vi "Mutex Attr Set Priority Ceiling.vi"(8 "error in (no error)":errorcluster, 10 "priority ceiling":i32, 11 "Mutex Attr in":T1) -> (0 "error out":errorcluster, 3 "Mutex Attr out":T1)   [LabVIEW 2013, in "Linux RT IPC.lvlib" / "POSIX Threads.lvlib" / "Mutex Attr.lvclass"]
doc: "Calls pthread_mutexattr_setprioceling() on the pthread mutex attribute object encapsulated by Mutex Attr.\n\nThis VI sets the priority ceiling for the provided mutex attribute object. The priority ceiling refers to the maximum priority that the mutex can be elevated to in the event of a priority inversion.\n\nRefer to online POSIX documentation for more information."
uses:
  Mutex Attr.lvclass
  Controls/reference.ctl
  POSIX Thread Object/POSIX Thread Object.lvclass/POSIX Thread Object.ctl
  POSIX Thread Object/Private VIs/libpthread path.vi
  POSIX Thread Object/Private VIs/get pthread error.vi
  POSIX Thread Object/POSIX Thread Object.lvclass
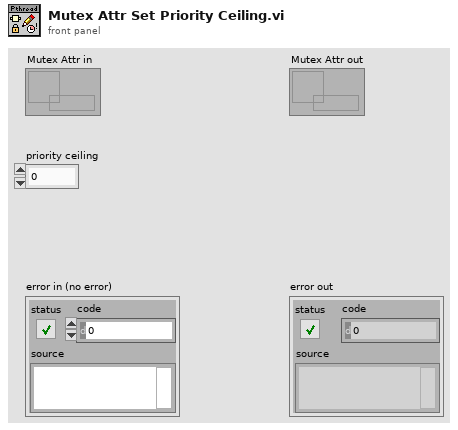
[diagram p1: front panel]
types:
  T1 = typedef "Linux RT IPC.lvlib/POSIX Threads.lvlib/Mutex Attr.lvclass/reference.ctl" = refnum<data-value>
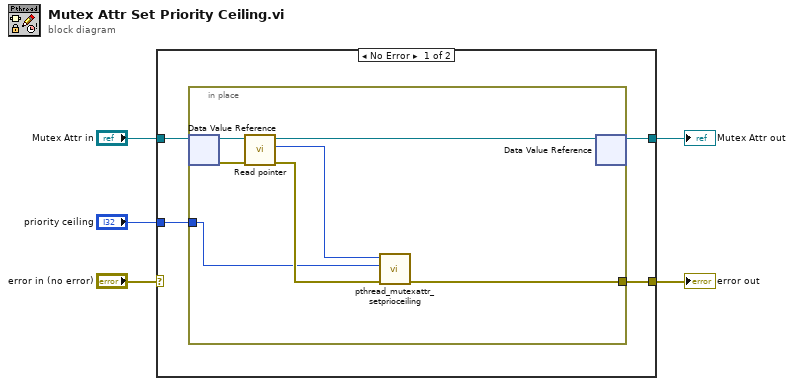
[diagram p0: block diagram]
diagram:
  n1 = case shown="No Error" "error in (no error)" {
    selector: "error in (no error)" -> [_ w18]
    tunnel: [w7 w18] -> w4
    tunnel: "Mutex Attr in" -> [w9 w17]
    tunnel: [w8 w17] -> w2
    tunnel: "priority ceiling" -> [w6 _]
    frame No Error {
      n2 = in-place {
        in-place-border: [w12] -> w7
        in-place-border: w6 -> [w10]
        n3 = in-place-dvr #1(w9) -> (w16:refnum<class "Mutex Attr.lvclass">, w14:errorcluster)
        n4 = call "Read pointer.vi"("error in (no error)"=w14, "POSIX Thread Object in"=w16) -> ("error out"=w13:errorcluster, "pointer"=w11:u64, "POSIX Thread Object out"=w15:refnum<class "Mutex Attr.lvclass">)  [unwired: 7 in]
        n5 = call "pthread_mutexattr_setprioceiling.vi"("error in (no error)"=w13, "priority ceiling"=w10, "mutex attr ptr in"=w11) -> ("error out"=w12:errorcluster)  [unwired: 7 in, 1 out]
        n6 = in-place-dvr #1(w15) -> (w8:T1)  [unwired: 1 out]
      }
    }
    frame Error {
    }
  }
  "Mutex Attr out" <- w2
  "error out" <- w4
